vi "TestFunction.vi"() -> ()   [LabVIEW 2018]
uses:
  Editor/Class/EditorThumbnail.lvclass
panel:
  in  "Next Button":bool
  in  "Previous Button":bool
  in  "Shadow":bool
  in  "Array":T1(array[cluster])
  out "index":u32
  in  "mouseState":enum16{"idle", "down", "move", "up"}(ring)
  out "Temp":cluster{"X":dbl[], "Y":sgl[]}[](graph)
  out "XY Graph":cluster{"Xdata":dbl[], "Ydata":sgl[]}[](graph)
  in  "add":bool
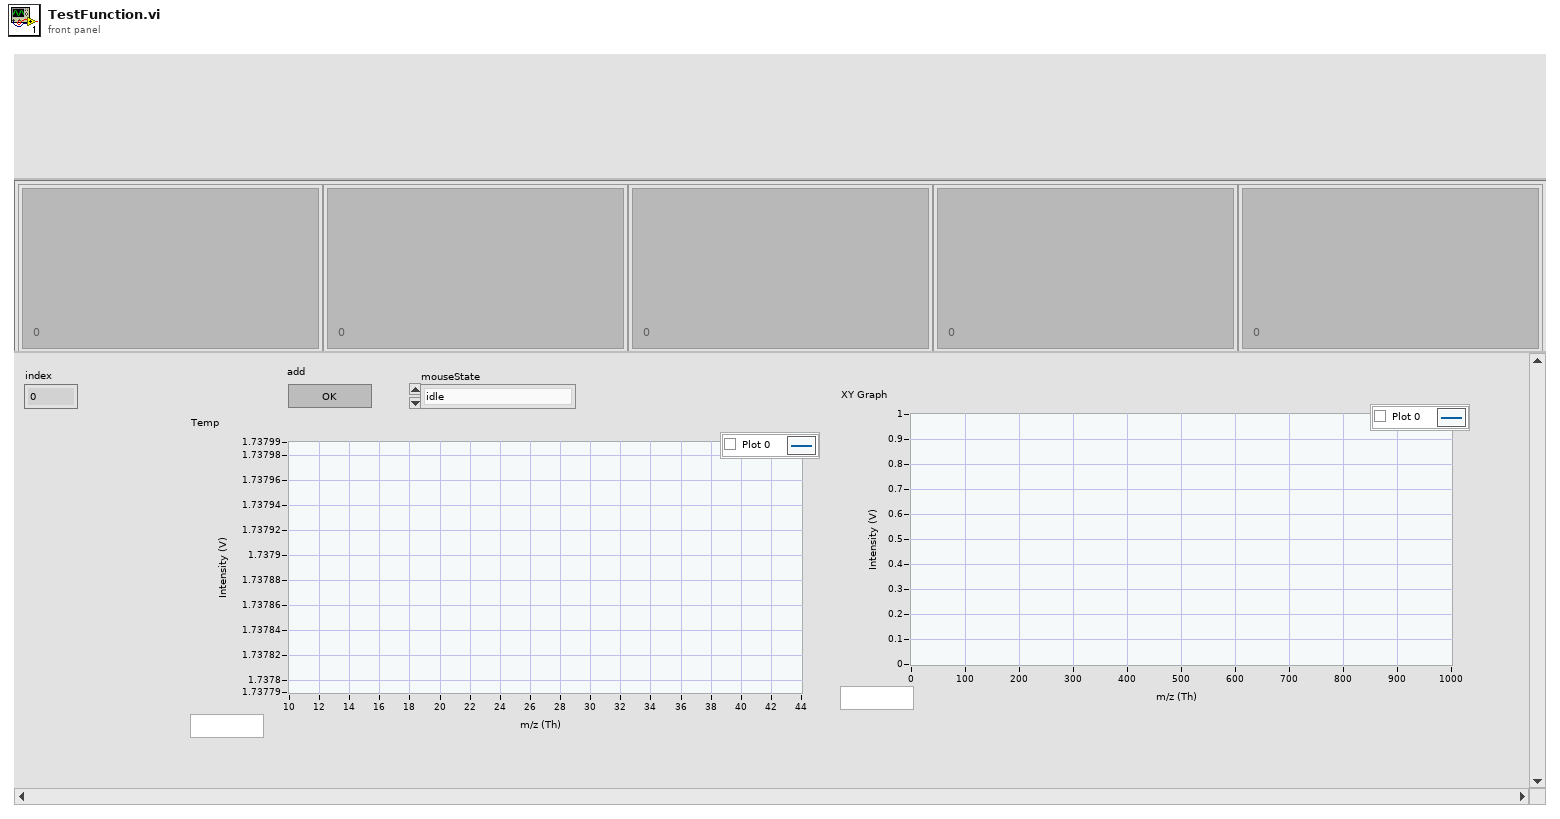
[diagram p1: front panel]
types:
  T1 = cluster{"index":u32, "data":cluster{"xdata":dbl[], "ydata":sgl[]}[], "peak":dbl[], "picture":picture}[]
  T2 = cluster{"graphRefnum":refnum<vi>, "shadowRefnum":refnum<vi>, "mouseState":refnum<vi>, "Previous Button":refnum<vi>, "Next Button":refnum<vi>, "thumbnailArrayRefnum":refnum<vi>, "topSpl":refnum<vi>, "bottomSpl":refnum<vi>}
  T3 = cluster{"plotIdx":i32, "Minimum":dbl, "Maximum":dbl}
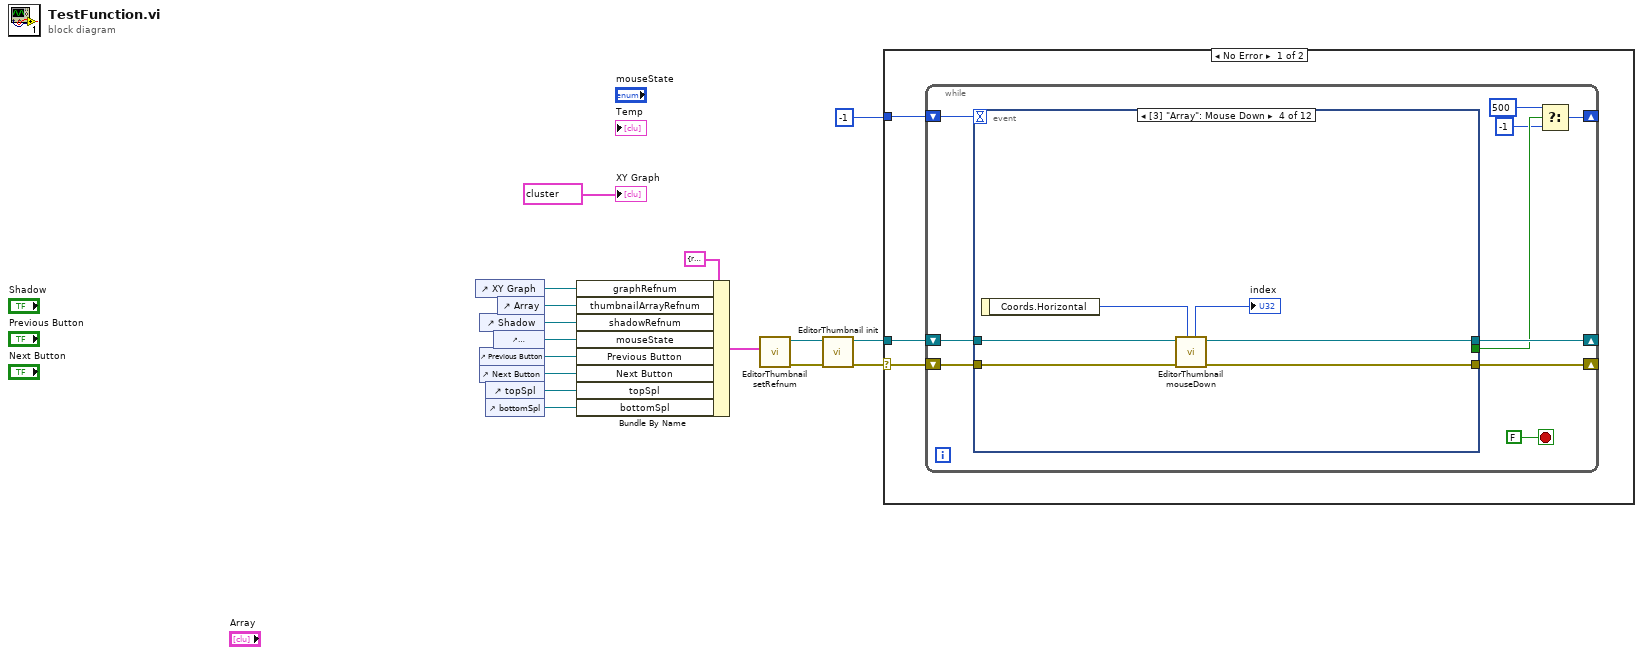
[diagram p0: block diagram]
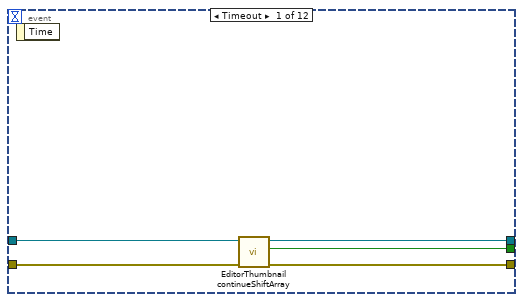
[diagram p2: hidden frame]
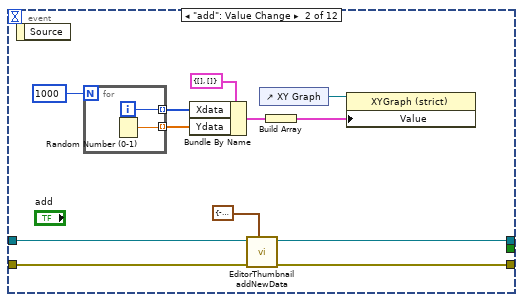
[diagram p3: hidden frame]
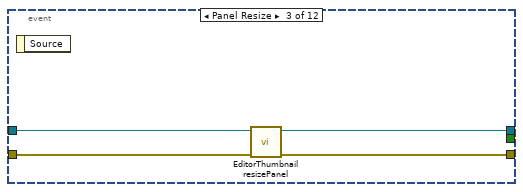
[diagram p4: hidden frame]
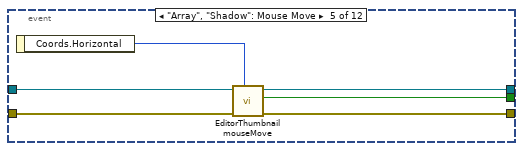
[diagram p5: hidden frame]
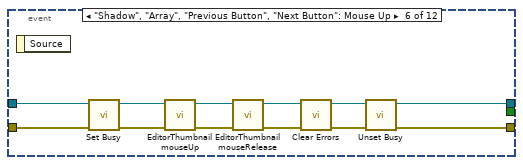
[diagram p6: hidden frame]
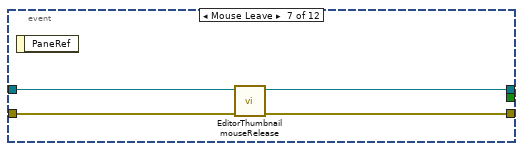
[diagram p7: hidden frame]
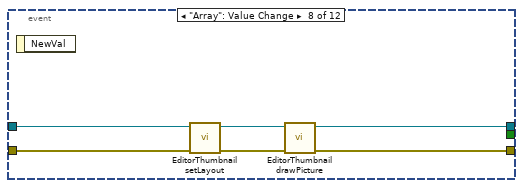
[diagram p8: hidden frame]
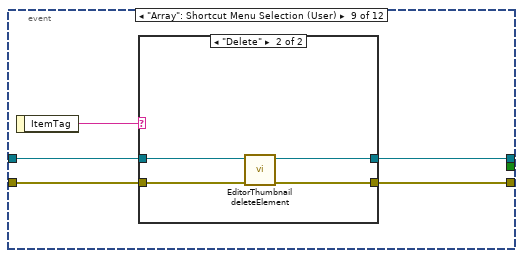
[diagram p9: hidden frame]
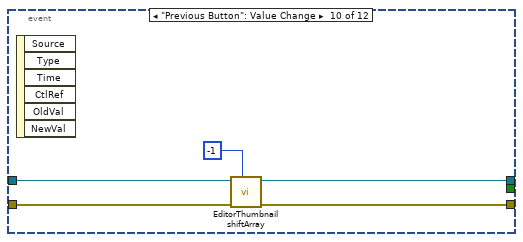
[diagram p11: hidden frame]
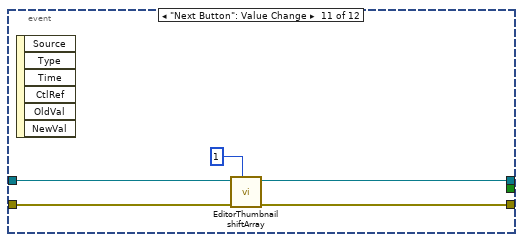
[diagram p12: hidden frame]
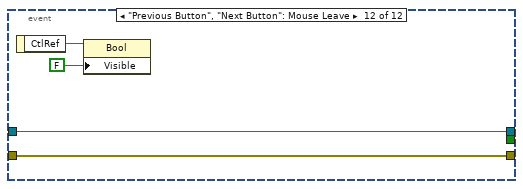
[diagram p13: hidden frame]
diagram:
  n1 = control-ref of="XY Graph"() -> (w11:refnum<vi>)
  n2 = control-ref of="Shadow"() -> (w10:refnum<vi>)
  n3 = control-ref of="Previous Button"() -> (w8:refnum<vi>)
  n4 = control-ref of="Next Button"() -> (w7:refnum<vi>)
  n5 = control-ref of="topSpl"() -> (w2:refnum<vi>)
  n6 = control-ref of="bottomSpl"() -> (w1:refnum<vi>)
  n7 = control-ref of="mouseState"() -> (w9:refnum<vi>)
  n8 = control-ref of="Array"() -> (w6:refnum<vi>)
  n9 = Bundle By Name(cluster=T2 {"graphRefnum"=refnum, "shadowRefnum"=refnum, "mouseState"=refnum, "Previous Button"=refnum, "Next Button"=refnum, "thumbnailArrayRefnum"=refnum, "topSpl"=refnum, "bottomSpl"=refnum} ("clusterRefnum"), "graphRefnum"=w11, "thumbnailArrayRefnum"=w6, "shadowRefnum"=w10, "mouseState"=w9, "Previous Button"=w8, "Next Button"=w7, "topSpl"=w2, "bottomSpl"=w1) -> (w3:T2)
  n10 = call "EditorThumbnail setRefnum.vi"("clusterRefnum"=w3) -> ("error out"=w14:errorcluster, "EditorThumbnail out"=w15:refnum<class "EditorThumbnail.lvclass">)  [unwired: 9 in]
  n11 = call "EditorThumbnail init.vi"("error in (no error)"=w14, "EditThumbnail in"=w15) -> ("error out"=w12:errorcluster, "EditThumbnail out"=w13:refnum<class "EditorThumbnail.lvclass">)  [unwired: 8 in]
  n12 = case shown="No Error" w12 {
    selector: w12 -> [w18 _]
    tunnel: w13 -> [w19 _]
    tunnel: -1 -> [w17 _]
    frame No Error {
      n13 = while {
        shift-right: [w26] -> _
        shift-left: w19 -> [w28]
        shift-right: [w24] -> _
        shift-left: w18 -> [w27]
        shift-right: [w20] -> _
        shift-left: w17 -> [w25]
        stop <- FALSE stop-if-true
        n14 = event shown="[3] \"Array\": Mouse Down" {
          selector: _ -> [_ _ _ _ _ _ _ _ _ _ _ _]
          dyn-events: _ -> [_ _ _ _ _ _ _ _ _ _ _ _]
          timeout: w25 -> [_ _ _ _ _ _ _ _ _ _ _ _]
          tunnel: w28 -> [w34 w46 w52 w58 w63 w73 w77 w83 w88 w98 w104 w108]
          tunnel: w27 -> [w33 w45 w51 w56 w62 w71 w76 w82 w87 w95 w103 w107]
          tunnel: [w31 w36 w49 w55 w61 w72 w75 w79 w85 w97 w101 w108] -> w26
          tunnel: [w32 w35 w50 w54 w60 w65 w74 w78 w86 w96 w100 w107] -> w24
          tunnel: [w30 _ _ _ w59 _ _ _ _ _ _ _] -> w23
          event Timeout {
            n15 = event-data() -> ()  [unwired: 1 in, 1 out]
            n16 = call "EditorThumbnail continueShiftArray.vi"("error in (no error)"=w33, "EditorThumbnail in"=w34) -> ("error out"=w32:errorcluster, "Timing"=w30:bool, "EditorThumbnail out"=w31:refnum<class "EditorThumbnail.lvclass">)  [unwired: 7 in]
          }
          event "add": Value Change {
            n17 = event-data() -> ()  [unwired: 1 in, 1 out]
            n18 = for {
              N: 1000 -> [_]
              tunnel: [w48] -> w42 mode=indexing
              tunnel: [w47] -> w43 mode=indexing
              i -> [w48]
              n19 = Random Number (0-1)() -> (number: 0 to 1=w47:dbl)
            }
            n20 = Bundle By Name(cluster=cluster{"Xdata":dbl[], "Ydata":sgl[]} {"Xdata"=[], "Ydata"=[]}, "Xdata"=w42, "Ydata"=w43) -> (w44:cluster{"Xdata":dbl[], "Ydata":sgl[]})
            n21 = call "EditorThumbnail addNewData.vi"("limit"=T3 {"plotIdx"=-1, "Minimum"=100.0, "Maximum"=900.0}, "error in (no error)"=w45, "EditorThumbnail in"=w46) -> ("error out"=w35:errorcluster, "EditorThumbnail out"=w36:refnum<class "EditorThumbnail.lvclass">)  [unwired: 7 in]
            n22 = control-ref of="XY Graph"() -> (w39:refnum<vi>)
            n23 = Build Array(w44) -> (w38:cluster{"Xdata":dbl[], "Ydata":sgl[]}[])
            n24 = property class="XYGraph (strict)"(reference=w39, "Value"=w38) -> ()  [unwired: 1 in, 2 out]
          }
          event Panel Resize {
            n25 = event-data() -> ()  [unwired: 1 in, 1 out]
            n26 = call "EditorThumbnail resizePanel.vi"("error in (no error)"=w51, "EditorThumbnail in"=w52) -> ("error out"=w50:errorcluster, "EditorThumbnail out"=w49:refnum<class "EditorThumbnail.lvclass">)  [unwired: 8 in]
          }
          event "Array": Mouse Down {
            n27 = event-data() -> ("Coords.Horizontal"=w57:i32)  [unwired: 1 in]
            n28 = call "EditorThumbnail mouseDown.vi"("coordsHorizontal"=w57, "error in (no error)"=w56, "EditorThumbnail in"=w58) -> ("error out"=w54:errorcluster, "EditorThumbnail out"=w55:refnum<class "EditorThumbnail.lvclass">, "index"=→"index":u32)  [unwired: 6 in]
          }
          event "Array", "Shadow": Mouse Move {
            n29 = event-data() -> ("Coords.Horizontal"=w64:i32)  [unwired: 1 in]
            n30 = call "EditorThumbnail mouseMove.vi"("coordsHorizontal"=w64, "error in (no error)"=w62, "EditorThumbnail in"=w63) -> ("error out"=w60:errorcluster, "Timing"=w59:bool, "EditorThumbnail out"=w61:refnum<class "EditorThumbnail.lvclass">)  [unwired: 6 in]
          }
          event "Shadow", "Array", "Previous Button", "Next Button": Mouse Up {
            n31 = event-data() -> ()  [unwired: 1 in, 1 out]
            n32 = call <vilib>:"Set Busy.vi"("error in (no error)"=w71) -> ("error out"=w70:errorcluster)  [unwired: 9 in, 1 out]
            n33 = call "EditorThumbnail mouseUp.vi"("error in (no error)"=w70, "EditorThumbnail in"=w73) -> ("error out"=w66:errorcluster, "EditorThumbnail out"=w67:refnum<class "EditorThumbnail.lvclass">)  [unwired: 8 in]
            n34 = call "EditorThumbnail mouseRelease.vi"("error in (no error)"=w66, "EditorThumbnail in"=w67) -> ("error out"=w69:errorcluster, "EditorThumbnail out"=w72:refnum<class "EditorThumbnail.lvclass">)  [unwired: 8 in]
            n35 = call <vilib>:"Clear Errors.vi"("error in (no error)"=w69) -> ("error out"=w68:errorcluster)  [unwired: 5 in, 1 out]
            n36 = call <vilib>:"Unset Busy.vi"("error in (no error)"=w68) -> ("error out"=w65:errorcluster)  [unwired: 10 in]
          }
          event Mouse Leave {
            n37 = event-data() -> ()  [unwired: 1 in, 1 out]
            n38 = call "EditorThumbnail mouseRelease.vi"("error in (no error)"=w76, "EditorThumbnail in"=w77) -> ("error out"=w74:errorcluster, "EditorThumbnail out"=w75:refnum<class "EditorThumbnail.lvclass">)  [unwired: 8 in]
          }
          event "Array": Value Change {
            n39 = event-data() -> ()  [unwired: 1 in, 1 out]
            n40 = call "EditorThumbnail setLayout.vi"("error in (no error)"=w82, "EditorThumbnail in"=w83) -> ("error out"=w80:errorcluster, "EditorThumbnail out"=w81:refnum<class "EditorThumbnail.lvclass">)  [unwired: 8 in]
            n41 = call "EditorThumbnail drawPicture.vi"("error in (no error)"=w80, "EditorThumbnail in"=w81) -> ("error out"=w78:errorcluster, "EditorThumbnail out"=w79:refnum<class "EditorThumbnail.lvclass">)  [unwired: 8 in]
          }
          event "Array": Shortcut Menu Selection (User) {
            n42 = event-data() -> ("ItemTag"=w84:string)  [unwired: 1 in]
            n43 = case shown="\"Delete\"" w84 {
              tunnel: w88 -> [w90 w94]
              tunnel: w87 -> [w89 w91]
              tunnel: [w89 w92] -> w86
              tunnel: [w90 w93] -> w85
              frame Default {
              }
              frame "Delete" {
                n44 = call "EditorThumbnail deleteElement.vi"("error in (no error)"=w91, "EditorThumbnail in"=w94) -> ("error out"=w92:errorcluster, "EditorThumbnail out"=w93:refnum<class "EditorThumbnail.lvclass">)  [unwired: 8 in]
              }
            }
          }
          event "Previous Button": Value Change {
            n45 = event-data() -> ()  [unwired: 1 in, 6 out]
            n46 = call "EditorThumbnail shiftArray.vi"("add"=-1, "error in (no error)"=w95, "EditorThumbnail in"=w98) -> ("error out"=w96:errorcluster, "EditorThumbnail out"=w97:refnum<class "EditorThumbnail.lvclass">)  [unwired: 7 in]
          }
          event "Next Button": Value Change {
            n47 = event-data() -> ()  [unwired: 1 in, 6 out]
            n48 = call "EditorThumbnail shiftArray.vi"("add"=1, "error in (no error)"=w103, "EditorThumbnail in"=w104) -> ("error out"=w100:errorcluster, "EditorThumbnail out"=w101:refnum<class "EditorThumbnail.lvclass">)  [unwired: 7 in]
          }
          event "Previous Button", "Next Button": Mouse Leave {
            n49 = event-data() -> ("CtlRef"=w106:refnum<vi>)  [unwired: 1 in]
            n50 = property class="Bool"(reference=w106, "Visible"=FALSE) -> ()  [unwired: 1 in, 2 out]
          }
        }
        n51 = Select(t=500, s=w23, f=-1) -> (s? t:f=w20:i32)
      }
    }
    frame Error {
    }
  }
  "XY Graph" <- cluster{"Xdata":dbl[], "Ydata":sgl[]}[] [{"Xdata"=array[1000 elements], "Ydata"=array[1000 elements]}] ("XY Graph")
